vi "init.vi"(8 "error in":errorcluster, 10 "TBM module configuration in":refnum<class "TBM module configuration.lvclass">, 11 "TDMS datalogger runtime in":refnum<class "TDMS datalogger runtime.lvclass">) -> (0 "error out":errorcluster, 1 "data allocations":T1, 2 "execution settings":T4, 3 "TDMS datalogger runtime out":refnum<class "TDMS datalogger runtime.lvclass">)   [LabVIEW 2015, in "TDMS datalogger runtime.lvclass"]
doc: "Provides an interface for initializing a module at runtime. While this interface performs no operations, a child should provide an override which may open any necessary references or sessions, allocate necessary memory, and perform any final configuration validataion before providing the full configuration <b>execution data</b> to the calling process."
uses:
  TDMS datalogger runtime.lvclass
  <vilib>/NI/Tag Bus Module Framework/module configuration/TBM module configuration.lvclass
  <vilib>/NI/Tag Bus Module Framework/runtime/execution settings.ctl
  <vilib>/NI/Tag Bus Module Framework/channel/data tables.ctl
  <vilib>/NI/Tag Bus/dictionary/data dictionary.lvclass
  <vilib>/NI/Tag Bus/dictionary table pair.ctl
  <vilib>/NI/Tag Bus/table/data table.ctl
  configuration/TDMS datalogger configuration.lvclass
  message to background process.ctl
  control enum.ctl
  response from background process.ctl
  response enum.ctl
  Logging Configuration.ctl
  configuration/Edge Direction.ctl
  <vilib>/NI/LogRotate/LogRotate.lvclass
  configuration/TDMS datalogger configuration.lvclass/TDMS datalogger configuration.ctl
  <vilib>/NI/Configuration Framework/serializable configuration/NISE_CEF_serializable configuration.lvclass/NISE_CEF_serializable configuration.ctl
  TDMS datalogger runtime.lvclass/TDMS datalogger runtime.ctl
  configuration/Read add enable channel.vi
  <vilib>/NI/Configuration Framework/serializable configuration/Read UID.vi
  configuration/Read queue size.vi
  configuration/Read Path.vi
  configuration/Read backup directory.vi
  configuration/Read log name.vi
  configuration/Read logrotate_options.vi
  configuration/Read Trigger Type.vi
  configuration/Read Pre-trigger Blocks.vi
  configuration/Read scans per write.vi
  configuration/Read Blocks to Log.vi
  configuration/Read Edge Direction.vi
  <vilib>/Utility/LVClass/Get LV Class Name.vi
  <vilib>/NI/Configuration Framework/error generator/NISE_error generator.vi
  <vilib>/NI/Tag Bus Module Framework/channel/TBM channel.lvclass
  <vilib>/NI/Tag Bus Module Framework/runtime/TBM module execution interface.lvclass
  <vilib>/NI/Tag Bus/table/data table.lvlib
  <vilib>/NI/Tag Bus/tag bus.lvlib
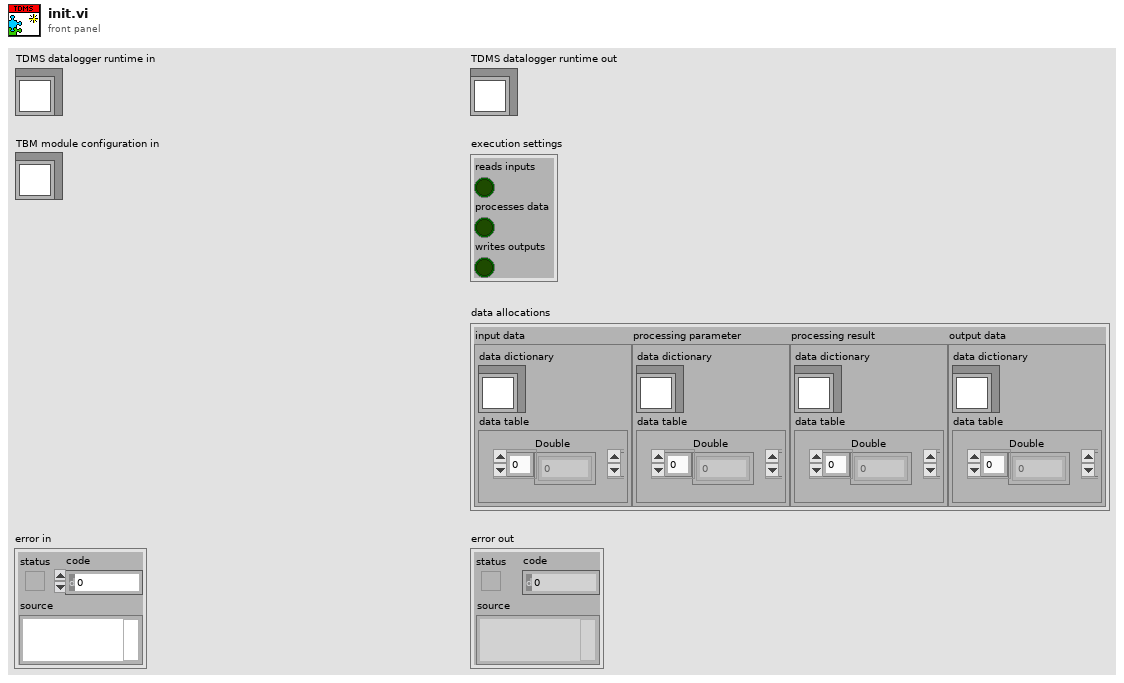
[diagram p1: front panel]
types:
  T1 = typedef "TBM channel.lvclass/data tables.ctl" = cluster{"input data":T2, "processing parameter":T2, "processing result":T2, "output data":T2}
  T2 = typedef "tag bus.lvlib/dictionary table pair.ctl" = cluster{"data dictionary":refnum<class "data dictionary.lvclass">, "data table":T3}
  T3 = typedef "tag bus.lvlib/data table.lvlib/data table.ctl" = cluster{"Double":dbl[], "Single":sgl[], "I64":i64[], "I32":i32[], "I16":i16[], "I8":i8[], "U64":u64[], "U32":u32[], "U16":u16[], "U8":u8[], "Boolean":bool[], "String":string[], "Array of Double":cluster{"DBL Array":dbl[]}[], "Array of Single":cluster{"SGL Array":sgl[]}[], "Array of I64":cluster{"I64 Array":i64[]}[], "Array of I32":cluster{"I32 Array":i32[]}[], "Array of I16":cluster{"I16 Array":i16[]}[], "Array of I8":cluster{"I8 Array":i8[]}[], "Array of U64":cluster{"U64 Array":u64[]}[], "Array of U32":cluster{"U32 Array":u32[]}[], "Array of U16":cluster{"U16 Array":u16[]}[], "Array of U8":cluster{"U8 Array":u8[]}[], "Array of Boolean":cluster{"Boolean Array":bool[]}[], "Array of String":cluster{"String Array":string[]}[]}
  T4 = typedef "TBM module execution interface.lvclass/execution settings.ctl" = cluster{"reads inputs":bool, "processes data":bool, "writes outputs":bool}
  T5 = typedef "TDMS datalogger runtime.lvclass/Logging Configuration.ctl" = cluster{"logging path":path, "backup directory":path, "group name":string, "scans per write":u16, "has enable channel":bool, "enable channel (bool)":i32, "has trigger channel":bool, "trigger channel (bool)":i32, "Blocks to log":i32, "Pre-trigger samples?":bool, "Edge Direction":T6, "LogRotate":refnum<class "LogRotate.lvclass">}
  T6 = typedef "TDMS datalogger configuration.lvclass/Edge Direction.ctl" = enum16{"Rising", "Falling"}
  T7 = cluster{"read mode":enum16{"polling", "blocking"}, "write mode":enum16{"polling", "blocking"}}
  T8 = typedef "TDMS datalogger runtime.lvclass/response from background process.ctl" = cluster{"response enum":T9, "datapack":refnum<data-value>, "error code":i32}
  T9 = typedef "TDMS datalogger runtime.lvclass/response enum.ctl" = enum16{"exit", "return buffer", "error"}
  T10 = typedef "TDMS datalogger runtime.lvclass/message to background process.ctl" = cluster{"control enum":T11, "datapack":refnum<data-value>, "Time Stamp":timestamp}
  T11 = typedef "TDMS datalogger runtime.lvclass/control enum.ctl" = enum16{"exit", "output data"}
  T12 = typedef "tag bus.lvlib/tag descriptor.lvclass/Data Type.ctl" = enum16{"Double", "Single", "I64", "I32", "I16", "I8", "U64", "U32", "U16", "U8", "Boolean", "String", "Array of Double", "Array of Single", "Array of I64", "Array of I32", "Array of I16", "Array of I8", "Array of U64", "Array of U32", "Array of U16", "Array of U8", "Array of Boolean", "Array of String"}
  T13 = typedef "LogRotate.lvclass/options.ctl" = cluster{"max file size (bytes)":i64, "rotate count":u32, "max age (days)":dbl, "No archive dir":bool, "Archive dir":path}
  T14 = typedef "TDMS datalogger configuration.lvclass/Trigger Type.ctl" = enum16{"None", "Start"}
  T15 = typedef "tag bus.lvlib/data dictionary.lvclass/full data dictionary.ctl" = cluster{"Double":string[], "Single":string[], "I64":string[], "I32":string[], "I16":string[], "I8":string[], "U64":string[], "U32":string[], "U16":string[], "U8":string[], "Boolean":string[], "String":string[], "Array of Double":string[], "Array of Single":string[], "Array of I64":string[], "Array of I32":string[], "Array of I16":string[], "Array of I8":string[], "Array of U64":string[], "Array of U32":string[], "Array of U16":string[], "Array of U8":string[], "Array of Boolean":string[], "Array of String":string[]}
  T16 = typedef "tag bus.lvlib/data table.lvlib/allocation specification.ctl" = cluster{"data type":T12, "size":i32}
  T17 = typedef "TDMS datalogger runtime.lvclass/data cache.ctl" = cluster{"timestamps":timestamp[], "Double":dbl[][], "Single":sgl[][], "I64":i64[][], "I32":i32[][], "I16":i16[][], "I8":i8[][], "U64":u64[][], "U32":u32[][], "U16":u16[][], "U8":u8[][], "Boolean":bool[][]}
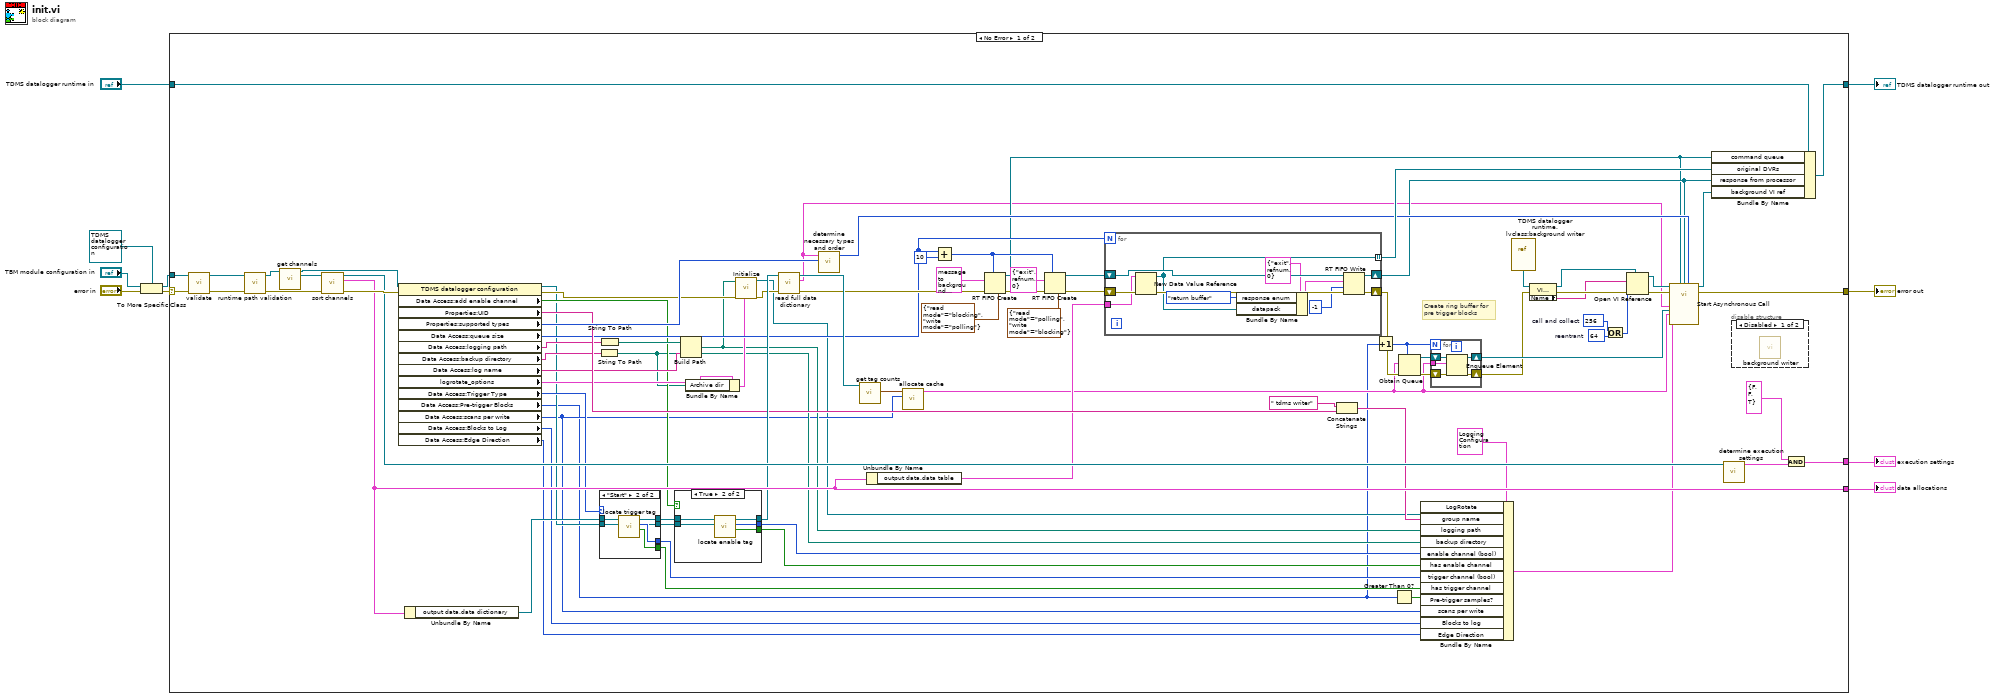
[diagram p0: block diagram]
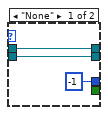
[diagram p2: hidden frame]
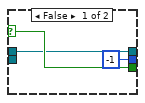
[diagram p3: hidden frame]
diagram:
  n1 = To More Specific Class(target class=refnum<class "TDMS datalogger configuration.lvclass"> refnum ("Synchronous module configuration"), reference="TBM module configuration in", error in="error in") -> (specific class reference=w9:refnum<class "TDMS datalogger configuration.lvclass">, error out=w10:errorcluster)
  n2 = case shown="No Error" w10 {
    selector: w10 -> [w92 w129]
    tunnel: w9 -> [w91 _]
    tunnel: "TDMS datalogger runtime in" -> [w90 w130]
    tunnel: [w89 w130] -> w4
    tunnel: [w79 w129] -> w3
    tunnel: [w78 _] -> w1
    tunnel: [w88 _] -> w2
    frame No Error {
      w83 = 64  # reentrant
      w82 = 256  # call and collect
      # "Create ring buffer for\npre trigger blocks"
      n3 = call-dynamic "validate.vi"("error in"=w92, "TDMS datalogger configuration in"=w91) -> ("error out"=w93:errorcluster, "TDMS datalogger configuration out"=w70:refnum<class "TDMS datalogger configuration.lvclass">)  [unwired: 8 in]
      n4 = call "runtime path validation.vi"("error in"=w93, "TDMS datalogger configuration in"=w70) -> ("error out"=w71:errorcluster, "TDMS datalogger configuration out"=w69:refnum<class "TDMS datalogger configuration.lvclass">)  [unwired: 8 in]
      n5 = call-dynamic "get channels.vi"("module configuration in"=w69) -> ("channels"=w67:refnum<class "TBM channel.lvclass">[], "module configuration out"=w68:refnum<class "TDMS datalogger configuration.lvclass">)  [unwired: 9 in]
      n6 = call <vilib>:"sort channels.vi"("error in"=w71, "channels in"=w67) -> ("error out"=w96:errorcluster, "data allocations"=w78:T1, "channels out"=w94:refnum<class "TBM channel.lvclass">[])  [unwired: 7 in]
      n7 = property class="TDMS datalogger configuration"(reference=w68, error in=w96) -> (reference out=w23:refnum<class "TDMS datalogger configuration.lvclass">, error out=w43:errorcluster, "Data Access:add enable channel"=w26:bool, "Properties:UID"=w73:string, "Properties:supported types"=w74:T12[], "Data Access:queue size"=w56:u16, "Data Access:logging path"=w47:string, "Data Access:backup directory"=w46:string, "Data Access:log name"=w45:string, "logrotate_options"=w42:T13, "Data Access:Trigger Type"=w24:T14, "Data Access:Pre-trigger Blocks"=w12:i32, "Data Access:scans per write"=w17:u16, "Data Access:Blocks to Log"=w19:i32, "Data Access:Edge Direction"=w16:T6)
      n8 = Unbundle By Name(w78) -> ("output data.data dictionary"=w27:refnum<class "data dictionary.lvclass">)
      n9 = String To Path(string=w46) -> (path=w18:path)
      n10 = String To Path(string=w47) -> (path=w44:path)
      n11 = case shown="\"Start\"" w24 {
        tunnel: w27 -> [w99 w104]
        tunnel: [w99 w103] -> w25
        tunnel: w23 -> [w98 w100]
        tunnel: [w98 w100] -> w22
        tunnel: [_ w102] -> w20
        tunnel: [-1 ("index") w101] -> w21
        frame "None" {
        }
        frame "Start" {
          n12 = call "locate trigger tag.vi"("TDMS datalogger configuration"=w100, "data dictionary in"=w104) -> ("found?"=w102:bool, "index"=w101:i32, "data dictionary out"=w103:refnum<class "data dictionary.lvclass">)  [unwired: 7 in]
        }
      }
      n13 = case shown="True" w26 {
        selector: w26 -> [w112 _]
        tunnel: w25 -> [w111 w113]
        tunnel: [w111 w117] -> w76
        tunnel: [w112 w115] -> w28
        tunnel: [-1 ("index") w116] -> w29
        tunnel: w22 -> [_ w114]
        frame False {
        }
        frame True {
          n14 = call "locate enable tag.vi"("TDMS datalogger configuration"=w114, "data dictionary in"=w113) -> ("found?"=w115:bool, "index"=w116:i32, "data dictionary out"=w117:refnum<class "data dictionary.lvclass">)  [unwired: 7 in]
        }
      }
      n15 = Build Path(base path=w44, name or relative path=w45) -> (appended path=w31:path)
      n16 = Bundle By Name(cluster=w42, "Archive dir"=w18) -> (w41:T13)
      n17 = call <vilib>:"Initialize.vi"("Options"=w41, "error in (no error)"=w43, "Log File Path"=w31) -> ("error out"=w40:errorcluster, "LogRotate"=w13:refnum<class "LogRotate.lvclass">)  [unwired: 7 in]
      n18 = call <vilib>:"read full data dictionary.vi"("error in"=w40, "data dictionary in"=w76) -> ("error out"=w65:errorcluster, "dictionary"=w36:T15, "data dictionary out"=w75:refnum<class "data dictionary.lvclass">)  [unwired: 7 in]
      n19 = call "determine necessary types and order.vi"("supported types"=w74, "dictionary"=w36) -> ("output type order"=w50:T12[])  [unwired: 9 in]
      n20 = call <vilib>:"get tag counts.vi"("data dictionary in"=w75) -> ("counts"=w86:T16[])  [unwired: 9 in, 1 out]
      n21 = Unbundle By Name(w78) -> ("output data.data table"=w66:T3)
      n22 = call "allocate cache.vi"("scans per write"=w17, "counts"=w86) -> ("cache allocation"=w33:T17)  [unwired: 9 in]
      n23 = Add(x=w56, y=u16 10) -> (x+y=w54:u16)
      n24 = RT FIFO Create(1:T10 {"control enum"=enum."exit", "datapack"=refnum, "Time Stamp"=timestamp(0 s since 1904-01-01)} ("message"), 3:w65, 4:w54, 7:T7 {"read mode"=enum."blocking", "write mode"=enum."polling"} ("r/w modes (polling,polling)")) -> (8:w48:refnum<k33>, 11:w64:errorcluster)  [unwired: 4 in, 1 out]
      n25 = RT FIFO Create(1:T8 {"response enum"=enum."exit", "datapack"=refnum, "error code"=0} ("message"), 3:w64, 4:w54, 7:T7 {"read mode"=enum."polling", "write mode"=enum."blocking"} ("r/w modes (polling,polling)")) -> (8:w57:refnum<k33>, 11:w61:errorcluster)  [unwired: 4 in, 1 out]
      n26 = for {
        N: w56 -> [_]
        shift-right: [w125] -> w39
        shift-left: w61 -> [w128]
        tunnel: w66 -> [w127]
        tunnel: [w119] -> w58 mode=indexing
        shift-right: [w124] -> w49
        shift-left: w57 -> [w123]
        n27 = New Data Value Reference(data value=w127, error in=w128) -> (data value reference=w119:refnum<data-value>, error out=w126:errorcluster)
        n28 = Bundle By Name(cluster=T8 {"response enum"=enum."exit", "datapack"=refnum, "error code"=0} ("element"), "response enum"=response_enum."return buffer", "datapack"=w119) -> (w120:T8)
        n29 = RT FIFO Write(0:w123, 1:w120, 2:-1 ("timeout in ms (0)"), 3:w126) -> (8:w124:refnum<k33>, 11:w125:errorcluster)  [unwired: 1 in, 2 out]
      }
      n30 = Concatenate Strings(" tdms writer" ("string"), w73) -> (w32:string)
      n31 = Increment(x=w12) -> (x+1=w11:i32)
      n32 = Greater Than 0?(x=w12) -> (x > 0?=w30:bool)
      n33 = Obtain Queue(max queue size (-1, unlimited)=w11, element data type=w33, error in (no error)=w39) -> (queue out=w37:refnum<queue>, error out=w38:errorcluster)  [unwired: 2 in, 1 out]
      n34 = Bundle By Name(cluster=T5 {"logging path"=path "", "backup directory"=path "", "group name"="", "scans per write"=0, "has enable channel"=FALSE, "enable channel (bool)"=0, "has trigger channel"=FALSE, "trigger channel (bool)"=0, "Blocks to log"=0, "Pre-trigger samples?"=FALSE, "Edge Direction"=enum."Rising", "LogRotate"=refnum} ("Logging Configuration"), "LogRotate"=w13, "group name"=w32, "logging path"=w31, "backup directory"=w18, "enable channel (bool)"=w29, "has enable channel"=w28, "trigger channel (bool)"=w21, "has trigger channel"=w20, "Pre-trigger samples?"=w30, "scans per write"=w17, "Blocks to log"=w19, "Edge Direction"=w16) -> (w34:T5)
      n35 = for {
        N: w11 -> [_]
        shift-right: [w106] -> w15
        shift-left: w37 -> [w107]
        shift-right: [w108] -> w14
        shift-left: w38 -> [w109]
        tunnel: w33 -> [w105]
        n36 = Enqueue Element(queue=w107, element=w105, error in (no error)=w109) -> (queue out=w106:refnum<queue>, error out=w108:errorcluster)  [unwired: 1 in, 1 out]
      }
      n37 = vi-ref "TDMS datalogger runtime.lvclass:background writer.vi"() -> (w53:refnum<vi>)
      n38 = property class="VI (strict)"(reference=w53, error in=w14) -> (reference out=w52:refnum<vi>, error out=w81:errorcluster, "Name"=w80:string)
      n39 = Or(x=w82, y=w83) -> (x .or. y?=w84:i32)
      n40 = Open VI Reference(type specifier VI Refnum (for type only)=w52, vi path=w80, options=w84, error in (no error)=w81) -> (vi reference=w51:refnum<vi>, error out=w85:errorcluster)  [unwired: 2 in]
      n41 = call-by-ref "Start Asynchronous Call"(reference=w51, error in=w85, "command queue"=w48, "response from processor"=w49, "output type order"=w50, "dictionary"=w36, "Ring Buffer"=w15, "cache allocation"=w33, "Logging Configuration"=w34) -> (reference out=w77:refnum<vi>, error out=w79:errorcluster)  [unwired: 8 in, 1 out]
      n42 = Bundle By Name(cluster=w90, "command queue"=w48, "original DVRs"=w58, "response from processor"=w49, "background VI ref"=w77) -> (w89:refnum<class "TDMS datalogger runtime.lvclass">)
      n43 = call <vilib>:"determine execution settings.vi"("channels"=w94) -> ("execution settings"=w95:T4)  [unwired: 10 in]
      n44 = disable-structure shown="Disabled" {
        frame Disabled {
          n45 = call "background writer.vi"() -> ()  [unwired: 15 in, 1 out]
        }
        frame Enabled {
        }
      }
      n46 = And(x=T4 {"reads inputs"=FALSE, "processes data"=FALSE, "writes outputs"=TRUE}, y=w95) -> (x .and. y?=w88:T4)
    }
    frame Error {
    }
  }
  "error out" <- w3
  "TDMS datalogger runtime out" <- w4
  "execution settings" <- w2
  "data allocations" <- w1
